vi "MQTT_Q_PVT_ReadFixedHeader.vi"(8 "error in":errorcluster, 10 "timeout ms (25000)":i32=25000, 11 "connection ID":refnum<k5>) -> (0 "error out":errorcluster, 1 "TimedOut":bool, 2 "Fixed Header":T1, 3 "connection ID out":refnum<k5>)   [LabVIEW 2015, in "MQTT_Q.lvclass"]
uses:
  MQTT_Q.lvclass
  MQTT_Q_PVT_FixedHeader.ctl
  MQTT_Q_PVT_MessageType.ctl
  MQTT_Q_QoS.ctl
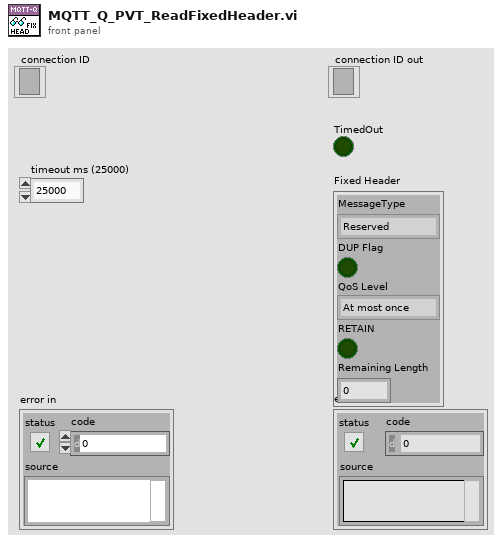
[diagram p1: front panel]
types:
  T1 = typedef "MQTT_Q.lvclass/MQTT_Q_PVT_FixedHeader.ctl" = cluster{"MessageType":T2, "DUP Flag":bool, "QoS Level":T3, "RETAIN":bool, "Remaining Length":u32}
  T2 = typedef "MQTT_Q.lvclass/MQTT_Q_PVT_MessageType.ctl" = enum32{"Reserved", "CONNECT", "CONNACK", "PUBLISH", "PUBACK", "PUBREC", "PUBREL", "PUBCOMP", "SUBSCRIBE", "SUBACK", "UNSUBSCRIBE", "UNSUBACK", "PINGREQ", "PINGRESP", "DISCONNECT", "Reserved2"}
  T3 = typedef "MQTT_Q.lvclass/MQTT_Q_QoS.ctl" = enum8{"At most once", "At least once", "Exactly once", "Reserved"}
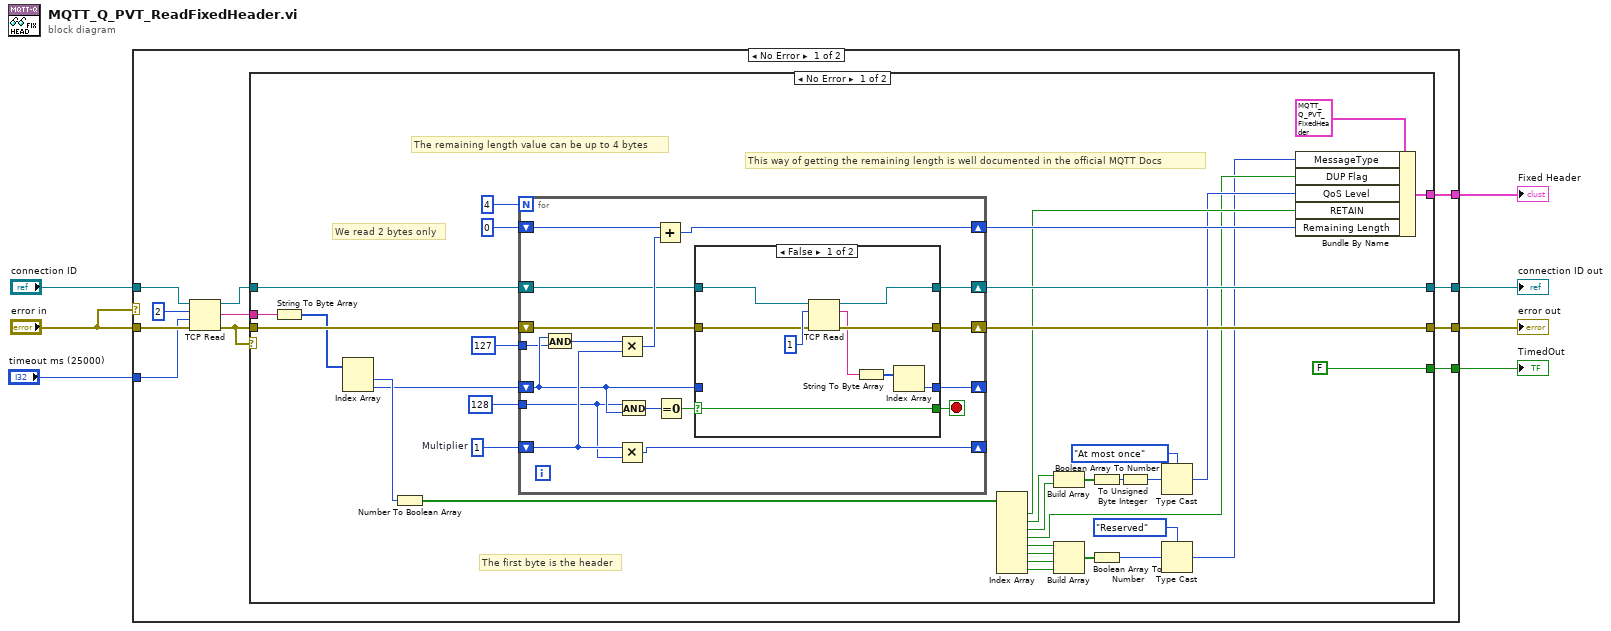
[diagram p0: block diagram]
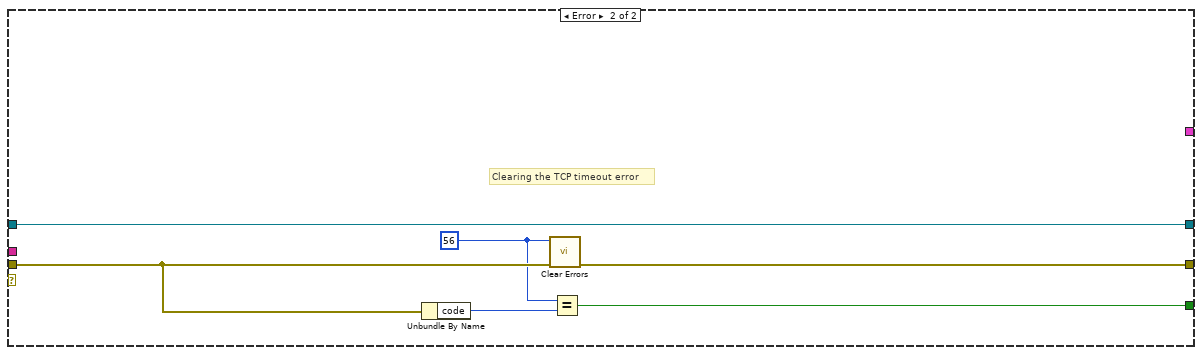
[diagram p3: hidden frame]
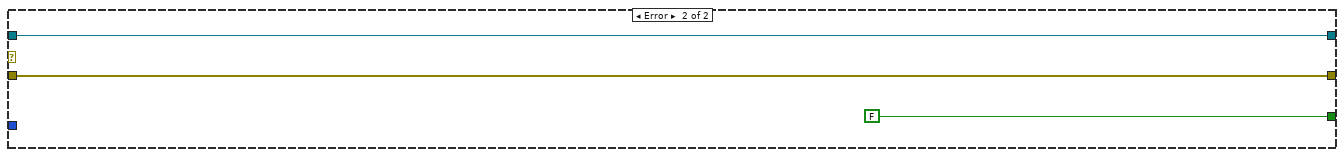
[diagram p4: hidden frame]
diagram:
  n1 = case shown="No Error" "error in" {
    tunnel: [w18 w91] -> w7
    tunnel: [w17 w92] -> w6
    tunnel: "connection ID" -> [w15 w92]
    tunnel: "error in" -> [w13 w91]
    tunnel: "timeout ms (25000)" -> [w11 _]
    tunnel: [w9 FALSE] -> w2
    tunnel: [w8 _] -> w1
    frame No Error {
      n2 = TCP Read(connection ID=w15, bytes to read=2, error in (no error)=w13, 9:w11) -> (connection ID out=w14:refnum<k5>, data out=w12:string, error out=w10:errorcluster)  [unwired: 1 in]
      n3 = case shown="No Error" w10 {
        tunnel: [w32 w88] -> w18
        tunnel: [w31 w89] -> w17
        tunnel: w14 -> [w30 w89]
        tunnel: w12 -> [w39 _]
        tunnel: w10 -> [w33 w87]
        tunnel: [FALSE w84] -> w9
        tunnel: [w21 _] -> w8
        frame No Error {
          w36 = u32 1  # Multiplier
          # "This way of getting the remaining length is well documented in the official MQTT Docs"
          # "The remaining length value can be up to 4 bytes"
          # "We read 2 bytes only"
          # "The first byte is the header"
          n4 = String To Byte Array(string=w39) -> (unsigned byte array=w19:u8[])
          n5 = Index Array(array=w19) -> (element #1=w52:u8, element #2=w20:u8)  [unwired: 2 in]
          n6 = Number To Boolean Array(number=w52) -> (Boolean array=w51:bool[])
          n7 = for {
            N: 4 -> [_]
            shift-right: [w70] -> _
            shift-left: w36 -> [w65]
            shift-right: [w66] -> w26
            shift-left: u32 0 -> [w68]
            shift-right: [w59] -> w32
            shift-left: w33 -> [w60]
            shift-right: [w58] -> _
            shift-left: w20 -> [w57]
            shift-right: [w56] -> w31
            shift-left: w30 -> [w61]
            tunnel: u8 127 -> [w55]
            tunnel: u32 128 ("y") -> [w54]
            stop <- w62 stop-if-true
            n8 = And(x=w57, y=w55) -> (x .and. y?=w69:u8)
            n9 = Multiply(x=w69, y=w65) -> (x*y=w67:u32)
            n10 = Multiply(x=w65, y=w54) -> (x*y=w70:u32)
            n11 = And(x=w54, y=w57) -> (x .and. y?=w64:u32)
            n12 = Add(x=w68, y=w67) -> (x+y=w66:u32)
            n13 = Equal To 0?(x=w64) -> (x = 0?=w63:bool)
            n14 = case shown="False" w63 {
              selector: w63 -> [w79 w83]
              tunnel: [w79 w83] -> w62
              tunnel: w61 -> [w78 w80]
              tunnel: w60 -> [w76 w82]
              tunnel: [w75 w82] -> w59
              tunnel: [w72 w81] -> w58
              tunnel: w57 -> [_ w81]
              tunnel: [w71 w80] -> w56
              frame False {
                n15 = TCP Read(connection ID=w78, bytes to read=1, error in (no error)=w76) -> (connection ID out=w71:refnum<k5>, data out=w74:string, error out=w75:errorcluster)  [unwired: 2 in]
                n16 = String To Byte Array(string=w74) -> (unsigned byte array=w73:u8[])
                n17 = Index Array(array=w73) -> (element=w72:u8)  [unwired: 1 in]
              }
              frame True {
              }
            }
          }
          n18 = Index Array(array=w51) -> (element #1=w25:bool, element #2=w50:bool, element #3=w49:bool, element #4=w23:bool, element #5=w47:bool, element #6=w46:bool, element #7=w45:bool, element #8=w44:bool)  [unwired: 8 in]
          n19 = Build Array(w50, w49) -> (w48:bool[])
          n20 = Build Array(w47, w46, w45, w44) -> (w43:bool[])
          n21 = Boolean Array To Number(Boolean array=w48) -> (number=w41:u32)
          n22 = Boolean Array To Number(Boolean array=w43) -> (number=w42:u32)
          n23 = To Unsigned Byte Integer(number=w41) -> (unsigned 8bit integer=w38:u8)
          n24 = Type Cast(type=MQTT_Q_QoS."At most once" ("QoS 2"), x=w38) -> (*(type *) &x=w24:T3)
          n25 = Type Cast(type=MQTT_Q_PVT_MessageType."Reserved" ("MessageType"), x=w42) -> (*(type *) &x=w22:T2)
          n26 = Bundle By Name(cluster=T1 {"MessageType"=enum."Reserved", "DUP Flag"=FALSE, "QoS Level"=enum."At most once", "RETAIN"=FALSE, "Remaining Length"=0} ("Fixed Header"), "MessageType"=w22, "DUP Flag"=w23, "QoS Level"=w24, "RETAIN"=w25, "Remaining Length"=w26) -> (w21:T1)
        }
        frame Error {
          w85 = 56 ("specific error code to clear (0: all)")
          # "Clearing the TCP timeout error"
          n27 = Unbundle By Name(w87) -> ("code"=w86:i32)
          n28 = call <vilib>:"Clear Errors.vi"("error in (no error)"=w87, "specific error code to clear (0: all)"=w85) -> ("error out"=w88:errorcluster)  [unwired: 4 in, 1 out]
          n29 = Equal?(x=w85, y=w86) -> (x = y?=w84:bool)
        }
      }
    }
    frame Error {
    }
  }
  "error out" <- w7
  "connection ID out" <- w6
  "TimedOut" <- w2
  "Fixed Header" <- w1
